vi "UI.vi"() -> ()   [LabVIEW 2019, in "Modules.lvlib" / "9226.lvclass"]
uses:
  9226.lvclass
  <vilib>/NI VeriStand/Custom Device API/Custom Device Item Ref.ctl
  9226 Configuration.ctl
  Supported RTD Types.ctl
  RSI Module/SubPanel Command.ctl
  RTD Rings for Type and Units.ctl
  RTD Coefficients.ctl
  C:/Users/nitest/Desktop/Git 2019/niveristand-scan-engine-module-libraries/Source/RSI Module/RSI Module.lvclass
  9226.lvclass/9226.ctl
  RSI Module/RSI Module.lvclass
  <vilib>/NI VeriStand/Custom Device API/Custom Device API.lvlib
panel:
  in  "_Measurement Units":u32(ring) items=["Raw Ohms", "Degrees Kelvin", "Degrees Celsius", "Degrees Fahrenheit", "Degrees Rankine"]
  in  "RTD Type":T1=2 items=["User Defined"=0, "TCR3750"=2, "TCR3851"=7]
  out "Selected Channel Settings Label":string="Selected Channel Settings"
  out "RTD Coefficients Label":string="RTD Coefficients"
  in  "Ro":dbl
  in  "C":dbl
  in  "B":dbl
  in  "A":dbl
  in  "RTD Type":T1=2 items=["User Defined"=0, "TCR3750"=2, "TCR3851"=7]
  in  "Measurement Units":u32(ring) items=["Raw Ohms", "Degrees Kelvin", "Degrees Celsius", "Degrees Fahrenheit", "Degrees Rankine"]
  in  "Channels":i32[](listbox)=[0]
  in  "SubPanel Event":refnum<user-event>
  in  "Header":cluster{"Section Name":string}={"Section Name"="NI 9205 Settings"}
  in  "Conversion Time":u32(ring) items=["200 ms", "2.5 ms"]
  in  "_9226 Config Data":T2 {"RTD_Type" items=["User Defined"=0, "TCR3750"=2, "TCR3851"=7]; "Degree Range" items=["Raw Ohms", "Degrees Kelvin", "Degrees Celsius", "Degrees Fahrenheit", "Degrees Rankine"]; "Conversion Time" items=["200 ms", "2.5 ms"]}
  in  "Node Ptr":T3 format="%.0x"
  in  "error in (no error)":errorcluster
  out "error out":errorcluster
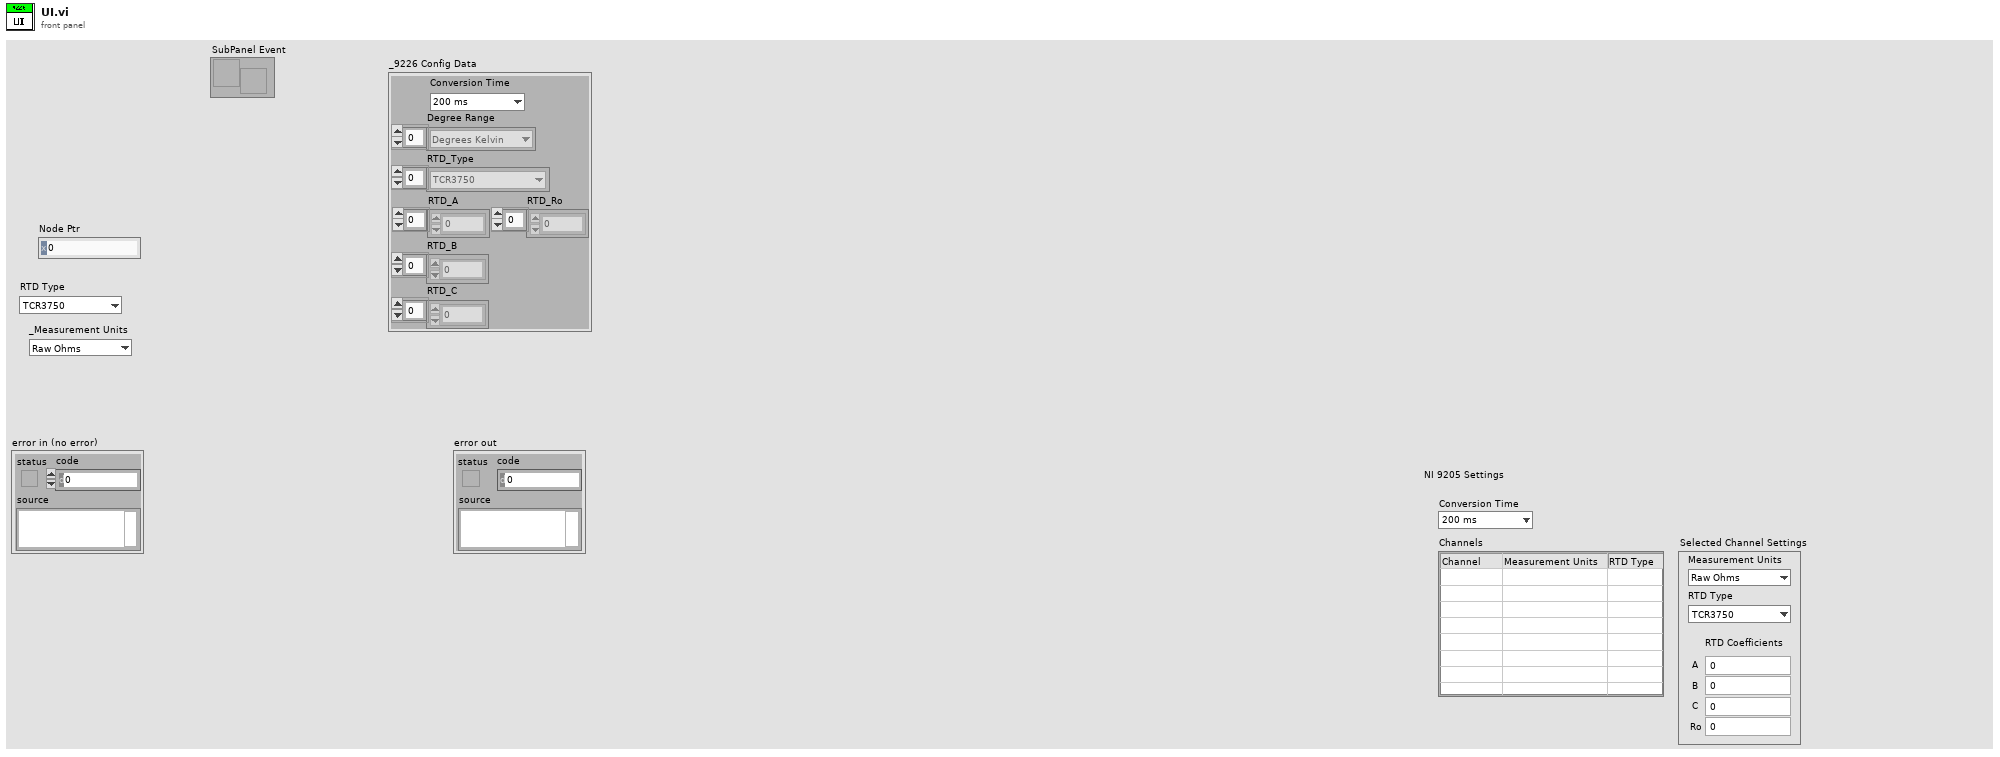
[diagram p1: front panel]
types:
  T1 = typedef "Modules.lvlib/9226.lvclass/Supported RTD Types.ctl" = u32
  T2 = typedef "Modules.lvlib/9226.lvclass/9226 Configuration.ctl" = cluster{"Conversion Time":u16, "Degree Range":u32[], "RTD_Type":T1[], "RTD_A":dbl[], "RTD_B":dbl[], "RTD_C":dbl[], "RTD_Ro":dbl[]}
  T3 = typedef "Custom Device API.lvlib/Custom Device Item Ref.ctl" = u64
  T4 = typedef "Modules.lvlib/9226.lvclass/RTD Rings for Type and Units.ctl" = cluster{"Type":refnum<vi>, "Units":refnum<vi>}
  T5 = typedef "Modules.lvlib/9226.lvclass/RTD Coefficients.ctl" = cluster{"A":refnum<vi>, "B":refnum<vi>, "C":refnum<vi>, "Ro":refnum<vi>}
  T6 = typedef "LVStringsAndValuesArrayTypeDef_U32.ctl" = cluster{"String":string, "Value":u32}[]
  T7 = typedef "Modules.lvlib/RSI Module.lvclass/Channels.ctl" = cluster{"# Input Channels":i32, "# Output Channels":i32, "Channel Type":T8, "Units":string}
  T8 = typedef "Modules.lvlib/RSI Module.lvclass/Channel Type.ctl" = enum16{"Analog", "Digital"}
  T9 = typedef "Modules.lvlib/RSI Module.lvclass/Module Models.ctl" = enum16{"Empty", "NI 9201", "NI 9203", "NI 9205", "NI 9206", "NI 9207", "NI 9208", "NI 9209", "NI 9210", "NI 9211", "NI 9212", "NI 9213", "NI 9214", "NI 9215", "NI 9216", "NI 9217", "NI 9219", "NI 9220", "NI 9221", "NI 9222", "NI 9223", "NI 9224", "NI 9225", "NI 9226", "NI 9227", "NI 9228", "NI 9229", "NI 9233", "NI 9234", "NI 9235", "NI 9236", "NI 9237", "NI 9239", "NI 9242", "NI 9244", "NI 9253", "NI 9263", "NI 9264", "NI 9265", "NI 9266", "NI 9269", "NI 9344", "NI 9350", "NI 9375", "NI 9401", "NI 9402", "NI 9403", "NI 9411", "NI 9421", "NI 9422", "NI 9423", "NI 9425", "NI 9426", "NI 9435", "NI 9436", "NI 9437", "NI 9472", "NI 9474", "NI 9475", "NI 9476", "NI 9477", "NI 9478", "NI 9481", "NI 9482", "NI 9485"}
  T10 = cluster{"Ohm degree range":u32, "RTD type":T1, "RTD user-defined A constant":dbl, "RTD user-defined B constant":dbl, "RTD user-defined C constant":dbl, "RTD user-defined Ro constant":dbl}[]
  T11 = cluster{"Ohm degree range":u32, "RTD type":T1, "RTD user-defined A constant":dbl, "RTD user-defined B constant":dbl, "RTD user-defined C constant":dbl, "RTD user-defined Ro constant":dbl}
  T12 = typedef "Modules.lvlib/RSI Module.lvclass/SubPanel Command.ctl" = enum16{"Stop"}
  T13 = typedef "Custom Device API.lvlib/Custom Device Channel.ctl" = cluster{"Type":T14, "Units":string, "Default Value":dbl, "Faultable":bool, "Scalable":bool}
  T14 = typedef "Custom Device API.lvlib/Custom Device Channel Type.ctl" = enum16{"Input", "Output"}
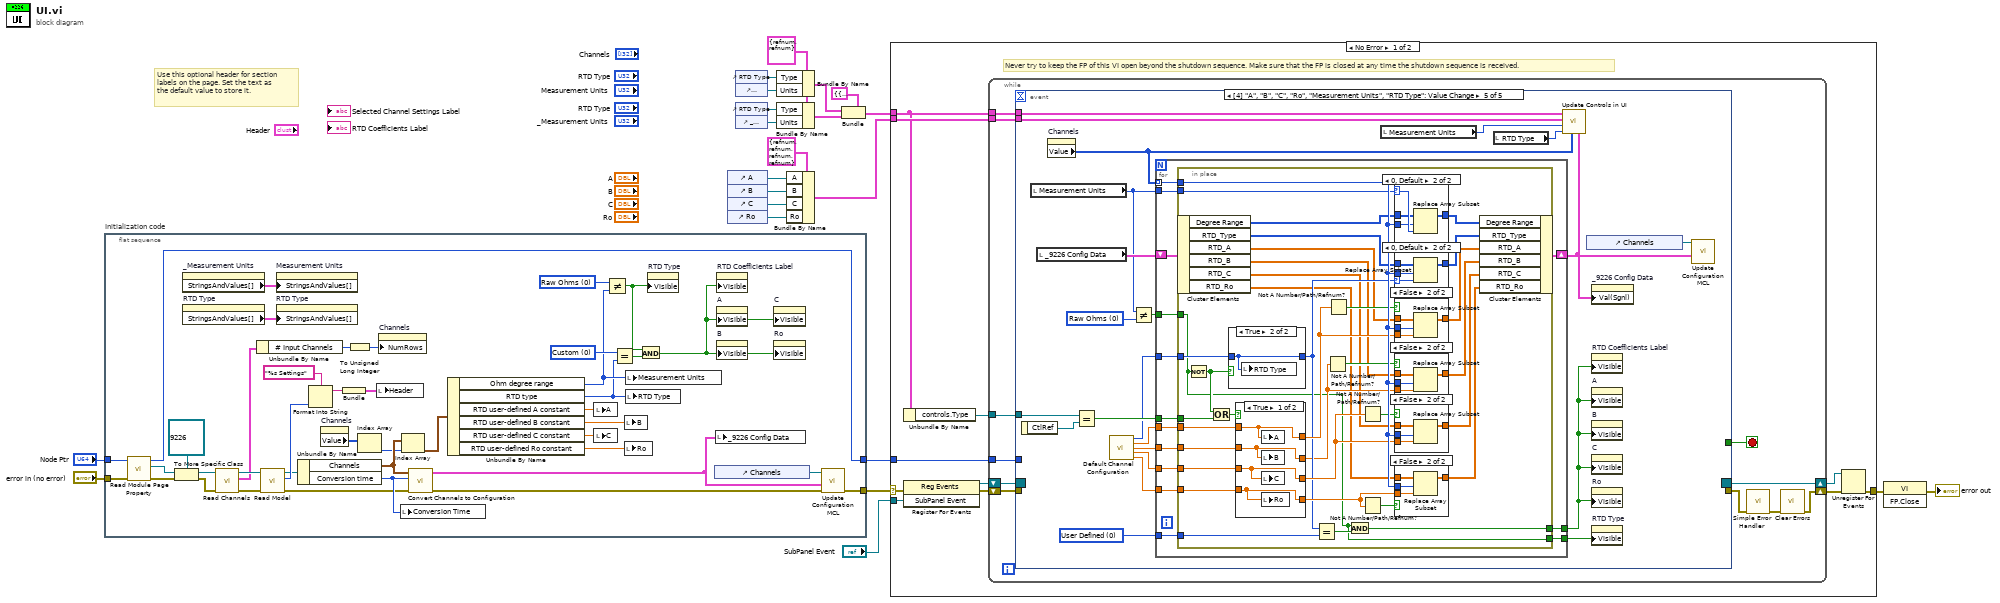
[diagram p0: block diagram]
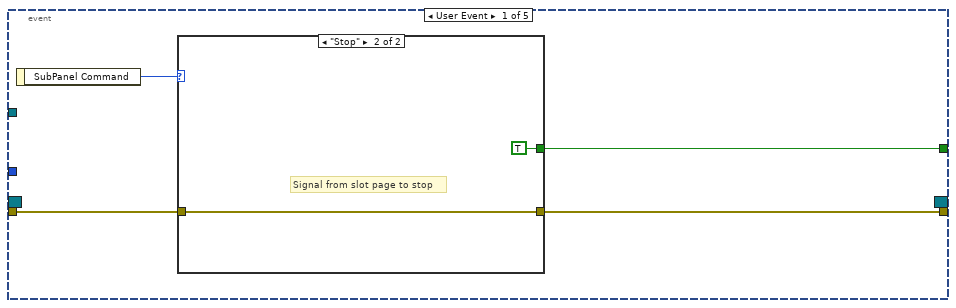
[diagram p2: hidden frame]
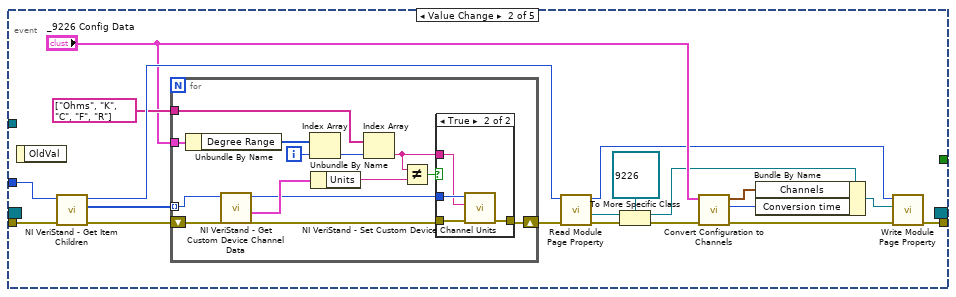
[diagram p4: hidden frame]
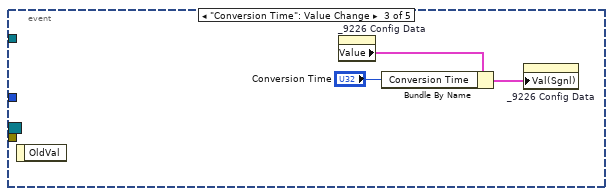
[diagram p6: hidden frame]
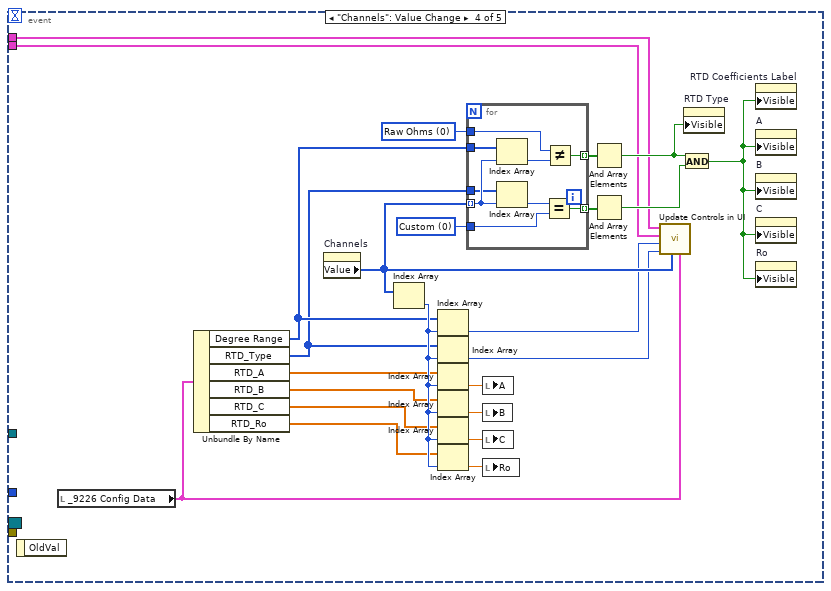
[diagram p7: hidden frame]
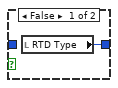
[diagram p8: hidden frame]
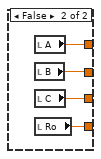
[diagram p9: hidden frame]
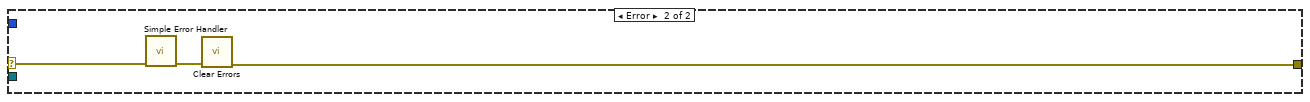
[diagram p16: hidden frame]
diagram:
  w13 = T4 {"Type"=refnum, "Units"=refnum} ("cluster")
  # "Use this optional header for section labels on the page. Set the text as the default value to store it."
  n1 = flat-sequence "Initialization code" {
    tunnel: "error in (no error)" -> [w62]
    tunnel: "Node Ptr" -> [w63]
    tunnel: [w49] -> w16
    tunnel: [w34] -> w19
    frame #0 {
      w46 = u32 0 items=["Raw Ohms", "Degrees Kelvin", "Degrees Celsius", "Degrees Fahrenheit", "Degrees Rankine"] ("Measurement Units")
      w47 = u32 0 items=["TCR3851"=1, "TCR3916"=3, "TCR3920"=4, "TCR3911"=5, "TCR3928"=6, "Custom"=0] ("RTD Type")
      n2 = call "Read Module Page Property.vi"("error in (no error)"=w62, "Node Ptr In"=w63) -> ("error out"=w61:errorcluster, "RSI Module"=w59:refnum<class "RSI Module.lvclass">, "Node Ptr Out"=w34:T3)  [unwired: 7 in]
      n3 = To More Specific Class(target class=refnum<class "9226.lvclass"> refnum ("9205 in"), reference=w59, error in=w61) -> (specific class reference=w40:refnum<class "9226.lvclass">, error out=w38:errorcluster)
      n4 = property on="_Measurement Units" class="Ring (strict)"() -> ("StringsAndValues[]"=w42:T6)  [unwired: 2 in, 2 out]
      n5 = property on="RTD Type" class="Ring (strict)"() -> ("StringsAndValues[]"=w41:T6)  [unwired: 2 in, 2 out]
      n6 = call "Read Channels.vi"("error in (no error)"=w38, "RSI Module in"=w40) -> ("error out"=w37:errorcluster, "Channels"=w36:T7, "RSI Module out"=w39:refnum<class "9226.lvclass">)  [unwired: 7 in]
      n7 = Unbundle By Name(w36) -> ("# Input Channels"=w35:i32)
      n8 = call "Read Model.vi"("error in (no error)"=w37, "RSI Module in"=w39) -> ("error out"=w52:errorcluster, "Model"=w57:T9, "RSI Module out"=w54:refnum<class "9226.lvclass">)  [unwired: 7 in]
      n9 = property on="Measurement Units" class="Ring (strict)"("StringsAndValues[]"=w42) -> ()  [unwired: 2 in, 2 out]
      n10 = property on="RTD Type" class="Ring (strict)"("StringsAndValues[]"=w41) -> ()  [unwired: 2 in, 2 out]
      n11 = Unbundle By Name(w54) -> ("Channels"=w32:T10, "Conversion time"=w53:u32)
      n12 = Format Into String(format string="%s Settings", w57) -> (resulting string=w55:string)  [unwired: 2 in, 1 out]
      n13 = property on="Channels" class="MCListbox (strict)"() -> ("Value"=w48:i32[])  [unwired: 2 in, 2 out]
      n14 = Bundle(w55) -> (w58:cluster{string})  [unwired: 1 in]
      n15 = To Unsigned Long Integer(number=w35) -> (unsigned 32bit integer=w23:u32)
      n16 = Index Array(array=w48) -> (element=w30:i32)  [unwired: 1 in]
      n17 = local write "Header"(w58) -> ()
      n18 = property on="Channels" class="MCListbox (strict)"("NumRows"=w23) -> ()  [unwired: 2 in, 2 out]
      n19 = local write "Conversion Time"(w53) -> ()
      n20 = Index Array(array=w32, index=w30) -> (element=w31:T11)
      n21 = call "Convert Channels to Configuration.vi"("error in"=w52, "Conversion time"=w53, "Channels"=w32) -> ("error out"=w50:errorcluster, "_9226 Config Data"=w33:T2)  [unwired: 7 in]
      n22 = Unbundle By Name(w31) -> ("Ohm degree range"=w29:u32, "RTD type"=w28:T1, "RTD user-defined A constant"=w27:dbl, "RTD user-defined B constant"=w26:dbl, "RTD user-defined C constant"=w25:dbl, "RTD user-defined Ro constant"=w24:dbl)
      n23 = local write "A"(w27) -> ()
      n24 = local write "C"(w25) -> ()
      n25 = Not Equal?(x=w46, y=w29) -> (x != y?=w44:bool)
      n26 = Equal?(x=w47, y=w28) -> (x = y?=w45:bool)
      n27 = local write "B"(w26) -> ()
      n28 = local write "Ro"(w24) -> ()
      n29 = local write "Measurement Units"(w29) -> ()
      n30 = local write "RTD Type"(w28) -> ()
      n31 = And(x=w44, y=w45) -> (x .and. y?=w43:bool)
      n32 = property on="RTD Type" class="Ring (strict)"("Visible"=w44) -> ()  [unwired: 2 in, 2 out]
      n33 = control-ref of="Channels"() -> (w51:refnum<vi>)
      n34 = local write "_9226 Config Data"(w33) -> ()
      n35 = property on="RTD Coefficients Label" class="Str"("Visible"=w43) -> ()  [unwired: 2 in, 2 out]
      n36 = property on="A" class="DigNum (strict)"("Visible"=w43) -> ()  [unwired: 2 in, 2 out]
      n37 = property on="B" class="DigNum (strict)"("Visible"=w43) -> ()  [unwired: 2 in, 2 out]
      n38 = property on="C" class="DigNum (strict)"("Visible"=w43) -> ()  [unwired: 2 in, 2 out]
      n39 = property on="Ro" class="DigNum (strict)"("Visible"=w43) -> ()  [unwired: 2 in, 2 out]
      n40 = call "Update Configuration MCL.vi"("error in"=w50, "_9226 Config"=w33, "_Channel Refnum"=w51) -> ("error out"=w49:errorcluster)  [unwired: 6 in]
    }
  }
  n41 = control-ref of="A"() -> (w8:refnum<vi>)
  n42 = control-ref of="B"() -> (w7:refnum<vi>)
  n43 = control-ref of="C"() -> (w6:refnum<vi>)
  n44 = control-ref of="Ro"() -> (w5:refnum<vi>)
  n45 = control-ref of="RTD Type"() -> (w15:refnum<vi>)
  n46 = control-ref of="Measurement Units"() -> (w14:refnum<vi>)
  n47 = control-ref of="RTD Type"() -> (w12:refnum<vi>)
  n48 = control-ref of="_Measurement Units"() -> (w11:refnum<vi>)
  n49 = Bundle By Name(cluster=w13, "Type"=w15, "Units"=w14) -> (w10:T4)
  n50 = Bundle By Name(cluster=w13, "Type"=w12, "Units"=w11) -> (w9:T4)
  n51 = Bundle By Name(cluster=T5 {"A"=refnum, "B"=refnum, "C"=refnum, "Ro"=refnum} ("RTD coefficients"), "A"=w8, "B"=w7, "C"=w6, "Ro"=w5) -> (w2:T5)
  n52 = Bundle(cluster=cluster{"controls":T4, "typedefs":T4} {"controls"={"Type"=refnum, "Units"=refnum}, "typedefs"={"Type"=refnum, "Units"=refnum}}, "controls"=w10, "typedefs"=w9) -> (w3:cluster{"controls":T4, "typedefs":T4})
  n53 = case shown="No Error" w16 {
    selector: w16 -> [w68 w280]
    tunnel: [w72 w278] -> w22
    tunnel: w19 -> [w69 _]
    tunnel: "SubPanel Event" -> [w67 _]
    tunnel: w3 -> [w65 _]
    tunnel: w2 -> [w66 _]
    frame No Error {
      # "Never try to keep the FP of this VI open beyond the shutdown sequence. Make sure that the FP is closed at any time the shutdown sequence is received."
      n54 = Unbundle By Name(w65) -> ("controls.Type"=w64:refnum<vi>)
      n55 = register-events(error in=w68, w67) -> (reference out=w70:refnum<event-registration>, error out=w71:errorcluster)  [unwired: 1 in]
      n56 = while {
        tunnel: w69 -> [w81]
        shift-right: [w78] -> w73
        shift-left: w71 -> [w84]
        shift-right: [w85] -> w74
        shift-left: w70 -> [w83]
        tunnel: w65 -> [w77]
        tunnel: w66 -> [w76]
        tunnel: w64 -> [w75]
        stop <- w82 stop-if-true
        n57 = event shown="[4] \"A\", \"B\", \"C\", \"Ro\", \"Measurement Units\", \"RTD Type\": Value Change" {
          selector: w83 -> [_ _ _ _ _]
          dyn-events: [_ _ _ _ _] -> w85
          timeout: _ -> [_ _ _ _ _]
          tunnel: w84 -> [w88 w102 _ _ _]
          tunnel: [w87 _ _ _ _] -> w82
          tunnel: [w86 w108 _ _ _] -> w80
          tunnel: w81 -> [_ w103 _ _ _]
          tunnel: w77 -> [_ _ _ w137 w182]
          tunnel: w76 -> [_ _ _ w135 w181]
          tunnel: w75 -> [_ _ _ _ w180]
          event User Event {
            n58 = event-data() -> ("SubPanel Command"=w89:T12)  [unwired: 1 out]
            n59 = case shown="\"Stop\"" w89 {
              tunnel: w88 -> [w90 w91]
              tunnel: [w90 w91] -> w86
              tunnel: [_ TRUE] -> w87
              frame Default {
              }
              frame "Stop" {
                # "Signal from slot page to stop"
              }
            }
          }
          event Value Change {
            n60 = event-data() -> ()  [unwired: 2 out]
            n61 = call <vilib>:"NI VeriStand - Get Item Children.vi"("error in (no error)"=w102, "Item Ref in"=w103) -> ("error out"=w101:errorcluster, "Child Refs"=w100:T3[], "Item Ref out"=w99:T3)  [unwired: 6 in, 1 out]
            n62 = for {
              tunnel: w100 -> [w117] mode=indexing
              shift-right: [w118] -> w98
              shift-left: w101 -> [w120]
              tunnel: "_9226 Config Data" -> [w125]
              tunnel: string[] ["Ohms", "K", "C", "F", "R"] -> [w124]
              i -> [w114]
              n63 = Unbundle By Name(w125) -> ("Degree Range"=w115:u32[])
              n64 = call <vilib>:"NI VeriStand - Get Custom Device Channel Data.vi"("error in (no error)"=w120, "Channel Ref in"=w117) -> ("error out"=w119:errorcluster, "Channel"=w122:T13, "Channel Ref out"=w116:T3)  [unwired: 4 in, 3 out]
              n65 = Index Array(array=w115, index=w114) -> (element=w113:u32)
              n66 = Unbundle By Name(w122) -> ("Units"=w121:string)
              n67 = Index Array(array=w124, index=w113) -> (element=w112:string)
              n68 = Not Equal?(x=w112, y=w121) -> (x != y?=w123:bool)
              n69 = case shown="True" w123 {
                tunnel: w116 -> [_ w130]
                tunnel: w112 -> [_ w129]
                tunnel: w119 -> [w126 w128]
                tunnel: [w126 w127] -> w118
                frame False {
                }
                frame True {
                  n70 = call <vilib>:"NI VeriStand - Set Custom Device Channel Units.vi"("error in (no error)"=w128, "Units"=w129, "Channel Ref in"=w130) -> ("error out"=w127:errorcluster)  [unwired: 7 in, 1 out]
                }
              }
            }
            n71 = call "Read Module Page Property.vi"("error in (no error)"=w98, "Node Ptr In"=w99) -> ("error out"=w109:errorcluster, "RSI Module"=w110:refnum<class "RSI Module.lvclass">, "Node Ptr Out"=w94:T3)  [unwired: 7 in]
            n72 = To More Specific Class(target class=refnum<class "9226.lvclass"> refnum ("9226"), reference=w110, error in=w109) -> (specific class reference=w93:refnum<class "9226.lvclass">, error out=w106:errorcluster)
            n73 = call "Convert Configuration to Channels.vi"("error in"=w106, "_9226 Config Data"="_9226 Config Data") -> ("error out"=w105:errorcluster, "Conversion Time"=w104:u32, "Channels"=w107:T10)  [unwired: 7 in]
            n74 = Bundle By Name(cluster=w93, "Channels"=w107, "Conversion time"=w104) -> (w95:refnum<class "9226.lvclass">)
            n75 = call "Write Module Page Property.vi"("error in (no error)"=w105, "RSI Module"=w95, "Node Ptr In"=w94) -> ("error out"=w108:errorcluster)  [unwired: 6 in, 2 out]
          }
          event "Conversion Time": Value Change {
            n76 = event-data() -> ()  [unwired: 2 out]
            n77 = property on="_9226 Config Data" class="Clust (strict)"() -> ("Value"=w133:T2)  [unwired: 2 in, 2 out]
            n78 = Bundle By Name(cluster=w133, "Conversion Time"="Conversion Time") -> (w131:T2)
            n79 = property on="_9226 Config Data" class="Clust (strict)"("Val(Sgnl)"=w131) -> ()  [unwired: 2 in, 2 out]
          }
          event "Channels": Value Change {
            w134 = u32 0 items=["TCR3851"=1, "TCR3750"=2, "TCR3916"=3, "TCR3920"=4, "TCR3911"=5, "TCR3928"=6, "Custom"=0] ("RTD Type")
            w136 = u32 0 items=["Raw Ohms", "Degrees Kelvin", "Degrees Celsius", "Degrees Fahrenheit", "Degrees Rankine"] ("Measurement Units")
            n80 = event-data() -> ()  [unwired: 2 out]
            n81 = local read "_9226 Config Data"() -> (w141:T2)
            n82 = Unbundle By Name(w141) -> ("Degree Range"=w148:u32[], "RTD_Type"=w147:T1[], "RTD_A"=w149:dbl[], "RTD_B"=w150:dbl[], "RTD_C"=w151:dbl[], "RTD_Ro"=w152:dbl[])
            n83 = property on="Channels" class="MCListbox (strict)"() -> ("Value"=w140:i32[])  [unwired: 2 in, 2 out]
            n84 = Index Array(array=w140) -> (element=w153:i32)  [unwired: 1 in]
            n85 = Index Array(array=w148, index=w153) -> (element=w138:u32)
            n86 = Index Array(array=w147, index=w153) -> (element=w139:T1)
            n87 = Index Array(array=w149, index=w153) -> (element=w157:dbl)
            n88 = Index Array(array=w150, index=w153) -> (element=w156:dbl)
            n89 = Index Array(array=w151, index=w153) -> (element=w155:dbl)
            n90 = Index Array(array=w152, index=w153) -> (element=w154:dbl)
            n91 = for {
              tunnel: w140 -> [w166] mode=indexing
              tunnel: w148 -> [w165]
              tunnel: w147 -> [w164]
              tunnel: [w161] -> w146 mode=indexing
              tunnel: [w160] -> w145 mode=indexing
              tunnel: w136 -> [w159]
              tunnel: w134 -> [w158]
              n92 = Index Array(array=w165, index=w166) -> (element=w163:u32)
              n93 = Index Array(array=w164, index=w166) -> (element=w162:T1)
              n94 = Equal?(x=w162, y=w158) -> (x = y?=w160:bool)
              n95 = Not Equal?(x=w159, y=w163) -> (x != y?=w161:bool)
            }
            n96 = local write "A"(w157) -> ()
            n97 = local write "B"(w156) -> ()
            n98 = local write "C"(w155) -> ()
            n99 = local write "Ro"(w154) -> ()
            n100 = And Array Elements(Boolean array=w146) -> (logical AND=w143:bool)
            n101 = And Array Elements(Boolean array=w145) -> (logical AND=w144:bool)
            n102 = call "Update Controls in UI.vi"("_9226 Config"=w141, "Values"=w140, "RTD Type"=w139, "Units"=w138, "RTD coefficients"=w135, "RTD types and units controls"=w137) -> ()  [unwired: 6 in]
            n103 = And(x=w143, y=w144) -> (x .and. y?=w142:bool)
            n104 = property on="RTD Type" class="Ring (strict)"("Visible"=w143) -> ()  [unwired: 2 in, 2 out]
            n105 = property on="RTD Coefficients Label" class="Str"("Visible"=w142) -> ()  [unwired: 2 in, 2 out]
            n106 = property on="A" class="DigNum (strict)"("Visible"=w142) -> ()  [unwired: 2 in, 2 out]
            n107 = property on="B" class="DigNum (strict)"("Visible"=w142) -> ()  [unwired: 2 in, 2 out]
            n108 = property on="C" class="DigNum (strict)"("Visible"=w142) -> ()  [unwired: 2 in, 2 out]
            n109 = property on="Ro" class="DigNum (strict)"("Visible"=w142) -> ()  [unwired: 2 in, 2 out]
          }
          event "A", "B", "C", "Ro", "Measurement Units": Value Change {
            w167 = T1 0 items=["User Defined"=0, "TCR3750"=2, "TCR3851"=7] ("y")
            w168 = u32 0 items=["Raw Ohms", "Degrees Kelvin", "Degrees Celsius", "Degrees Fahrenheit", "Degrees Rankine"] ("Measurement Units")
            n110 = event-data() -> ("CtlRef"=w185:refnum<vi>)  [unwired: 1 out]
            n111 = local read "Measurement Units"() -> (w171:u32)
            n112 = local read "_9226 Config Data"() -> (w177:T2)
            n113 = property on="Channels" class="MCListbox (strict)"() -> ("Value"=w186:i32[])  [unwired: 2 in, 2 out]
            n114 = Equal?(x=w180, y=w185) -> (x = y?=w184:bool)
            n115 = call "Default Channel Configuration.vi"() -> ("RTD type"=w176:T1, "RTD_A"=w175:dbl, "RTD_B"=w174:dbl, "RTD_C"=w173:dbl, "RTD_Ro"=w172:dbl)  [unwired: 9 in, 2 out]
            n116 = Not Equal?(x=w171, y=w168) -> (x != y?=w170:bool)
            n117 = for {
              tunnel: w186 -> [w201] mode=indexing
              tunnel: w184 -> [w202]
              tunnel: [w200] -> w179
              shift-right: [w191] -> w178
              shift-left: w177 -> [w192]
              tunnel: w176 -> [w199]
              tunnel: w175 -> [w198]
              tunnel: w174 -> [w197]
              tunnel: w173 -> [w196]
              tunnel: w172 -> [w195]
              tunnel: w170 -> [w193]
              tunnel: w171 -> [w194]
              tunnel: [w190] -> w169
              tunnel: w167 -> [w189]
              n118 = in-place {
                in-place-border: w202 -> [w237]
                in-place-border: w201 -> [w235]
                in-place-border: [w224] -> w200
                in-place-border: w199 -> [w223]
                in-place-border: w198 -> [w222]
                in-place-border: w197 -> [w221]
                in-place-border: w196 -> [w220]
                in-place-border: w195 -> [w219]
                in-place-border: w194 -> [w218]
                in-place-border: w193 -> [w204]
                in-place-border: [w204] -> w190
                in-place-border: w189 -> [w203]
                n119 = in-place-cluster #1(w192) -> ("Degree Range"=w211:u32[], "RTD_Type"=w212:T1[], "RTD_A"=w213:dbl[], "RTD_B"=w214:dbl[], "RTD_C"=w215:dbl[], "RTD_Ro"=w216:dbl[])
                n120 = Not(x=w204) -> (.not. x?=w227:bool)
                n121 = Or(x=w227, y=w237) -> (x .or. y?=w236:bool)
                n122 = case shown="True" w227 {
                  tunnel: [w238 w239] -> w226
                  tunnel: w223 -> [_ w239]
                  frame False {
                    n123 = local read "RTD Type"() -> (w238:T1)
                  }
                  frame True {
                    n124 = local write "RTD Type"(w239) -> ()
                  }
                }
                n125 = case shown="True" w236 {
                  tunnel: w222 -> [w243 _]
                  tunnel: w221 -> [w242 _]
                  tunnel: w220 -> [w241 _]
                  tunnel: w219 -> [w240 _]
                  tunnel: [w243 w247] -> w229
                  tunnel: [w242 w246] -> w217
                  tunnel: [w241 w245] -> w231
                  tunnel: [w240 w244] -> w233
                  frame True {
                    n126 = local write "A"(w243) -> ()
                    n127 = local write "B"(w242) -> ()
                    n128 = local write "C"(w241) -> ()
                    n129 = local write "Ro"(w240) -> ()
                  }
                  frame False {
                    n130 = local read "A"() -> (w247:dbl)
                    n131 = local read "B"() -> (w246:dbl)
                    n132 = local read "C"() -> (w245:dbl)
                    n133 = local read "Ro"() -> (w244:dbl)
                  }
                }
                n134 = Equal?(x=w226, y=w203) -> (x = y?=w225:bool)
                n135 = Not A Number/Path/Refnum?(number/path/refnum=w217) -> (NaN/Path/Refnum?=w230:bool)
                n136 = Not A Number/Path/Refnum?(number/path/refnum=w229) -> (NaN/Path/Refnum?=w228:bool)
                n137 = And(x=w204, y=w225) -> (x .and. y?=w224:bool)
                n138 = Not A Number/Path/Refnum?(number/path/refnum=w231) -> (NaN/Path/Refnum?=w232:bool)
                n139 = Not A Number/Path/Refnum?(number/path/refnum=w233) -> (NaN/Path/Refnum?=w234:bool)
                n140 = case shown="0, Default" w218 {
                  selector: w218 -> [_ w276]
                  tunnel: [w273 w277] -> w210
                  tunnel: w211 -> [w273 w275]
                  tunnel: w235 -> [_ w274]
                  frame 99 {
                  }
                  frame 0, Default {
                    n141 = Replace Array Subset(array=w275, new element=w276, index=w274) -> (w277:u32[])
                  }
                }
                n142 = case shown="0, Default" w226 {
                  selector: w226 -> [_ w271]
                  tunnel: [w268 w272] -> w209
                  tunnel: w212 -> [w268 w270]
                  tunnel: w235 -> [_ w269]
                  frame 99 {
                  }
                  frame 0, Default {
                    n143 = Replace Array Subset(array=w270, new element=w271, index=w269) -> (w272:T1[])
                  }
                }
                n144 = case shown="False" w228 {
                  tunnel: [w263 w267] -> w208
                  tunnel: w213 -> [w263 w266]
                  tunnel: w235 -> [_ w265]
                  tunnel: w229 -> [_ w264]
                  frame True {
                  }
                  frame False {
                    n145 = Replace Array Subset(array=w266, new element=w264, index=w265) -> (w267:dbl[])
                  }
                }
                n146 = case shown="False" w230 {
                  tunnel: [w258 w262] -> w207
                  tunnel: w214 -> [w258 w261]
                  tunnel: w235 -> [_ w260]
                  tunnel: w217 -> [_ w259]
                  frame True {
                  }
                  frame False {
                    n147 = Replace Array Subset(array=w261, new element=w259, index=w260) -> (w262:dbl[])
                  }
                }
                n148 = case shown="False" w232 {
                  tunnel: [w253 w257] -> w206
                  tunnel: w215 -> [w253 w256]
                  tunnel: w235 -> [_ w255]
                  tunnel: w231 -> [_ w254]
                  frame True {
                  }
                  frame False {
                    n149 = Replace Array Subset(array=w256, new element=w254, index=w255) -> (w257:dbl[])
                  }
                }
                n150 = case shown="False" w234 {
                  tunnel: [w248 w252] -> w205
                  tunnel: w216 -> [w248 w251]
                  tunnel: w235 -> [_ w250]
                  tunnel: w233 -> [_ w249]
                  frame True {
                  }
                  frame False {
                    n151 = Replace Array Subset(array=w251, new element=w249, index=w250) -> (w252:dbl[])
                  }
                }
                n152 = in-place-cluster #1("Degree Range"=w210, "RTD_Type"=w209, "RTD_A"=w208, "RTD_B"=w207, "RTD_C"=w206, "RTD_Ro"=w205) -> (w191:T2)
              }
            }
            n153 = local read "Measurement Units"() -> (w188:u32)
            n154 = local read "RTD Type"() -> (w187:T1)
            n155 = call "Update Controls in UI.vi"("_9226 Config"=w178, "Values"=w186, "RTD Type"=w187, "Units"=w188, "RTD coefficients"=w181, "RTD types and units controls"=w182) -> ()  [unwired: 6 in]
            n156 = control-ref of="Channels"() -> (w183:refnum<vi>)
            n157 = property on="_9226 Config Data" class="Clust (strict)"("Val(Sgnl)"=w178) -> ()  [unwired: 2 in, 2 out]
            n158 = property on="RTD Coefficients Label" class="Str"("Visible"=w179) -> ()  [unwired: 2 in, 2 out]
            n159 = property on="A" class="DigNum (strict)"("Visible"=w179) -> ()  [unwired: 2 in, 2 out]
            n160 = property on="B" class="DigNum (strict)"("Visible"=w179) -> ()  [unwired: 2 in, 2 out]
            n161 = property on="C" class="DigNum (strict)"("Visible"=w179) -> ()  [unwired: 2 in, 2 out]
            n162 = property on="Ro" class="DigNum (strict)"("Visible"=w179) -> ()  [unwired: 2 in, 2 out]
            n163 = property on="RTD Type" class="Ring (strict)"("Visible"=w169) -> ()  [unwired: 2 in, 2 out]
            n164 = call "Update Configuration MCL.vi"("_9226 Config"=w178, "_Channel Refnum"=w183) -> ()  [unwired: 7 in, 1 out]
          }
        }
        n165 = call <vilib>:"Simple Error Handler.vi"("error in (no error)"=w80) -> ("error out"=w79:errorcluster)  [unwired: 1 in, 7 out]
        n166 = call <vilib>:"Clear Errors.vi"("error in (no error)"=w79) -> ("error out"=w78:errorcluster)  [unwired: 1 in, 5 out]
      }
      n167 = Unregister For Events(event registration refnum=w74, error in=w73) -> (error out=w72:errorcluster)
    }
    frame Error {
      n168 = call <vilib>:"Simple Error Handler.vi"("error in (no error)"=w280) -> ("error out"=w279:errorcluster)  [unwired: 1 in, 7 out]
      n169 = call <vilib>:"Clear Errors.vi"("error in (no error)"=w279) -> ("error out"=w278:errorcluster)  [unwired: 1 in, 5 out]
    }
  }
  n170 = invoke class="VI" method="FP.Close"(error in=w22) -> (error out=→"error out":errorcluster)  [unwired: 2 in, 2 out]
